vi "Take photo.vi"() -> ()   [LabVIEW 2020]
uses:
  <vilib>/userDefined/High Color/IMAQdx.ctl
  <vilib>/vision/driver/NI_Vision_Acquisition_Software.lvlib
  <vilib>/vision/NI_Vision_Development_Module.lvlib
panel:
  out "Number of Matches":i32
  out "error out":errorcluster
  out "Image 2":T1(plugin-control)
  in  "Parameters":T2={"Number of Matches Requested"=1, "Minimum Match Score"=800.0, "Angle Ranges"=[]}
  in  "File Path":path
  out "Image":T1(plugin-control)
  in  "stop":bool
  in  "Session In":T3
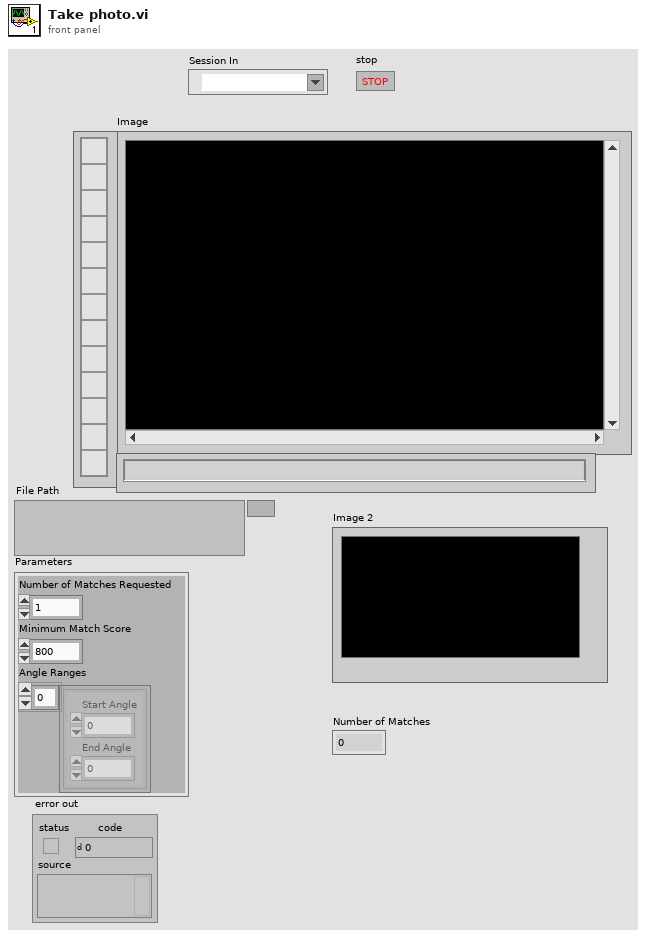
[diagram p1: front panel]
types:
  T1 = typedef "IMAQ Image.ctl" = refnum<image>
  T2 = cluster{"Number of Matches Requested":i32, "Minimum Match Score":sgl, "Angle Ranges":cluster{"Start Angle":sgl, "End Angle":sgl}[]}
  T3 = typedef "IMAQdx.ctl" = refnum<k21>
  T4 = cluster{"Position":cluster{"x":sgl, "y":sgl}, "Angle":sgl, "Scale":sgl, "Score":sgl, "Bounding Box":cluster{"x":sgl, "y":sgl}[]}[]
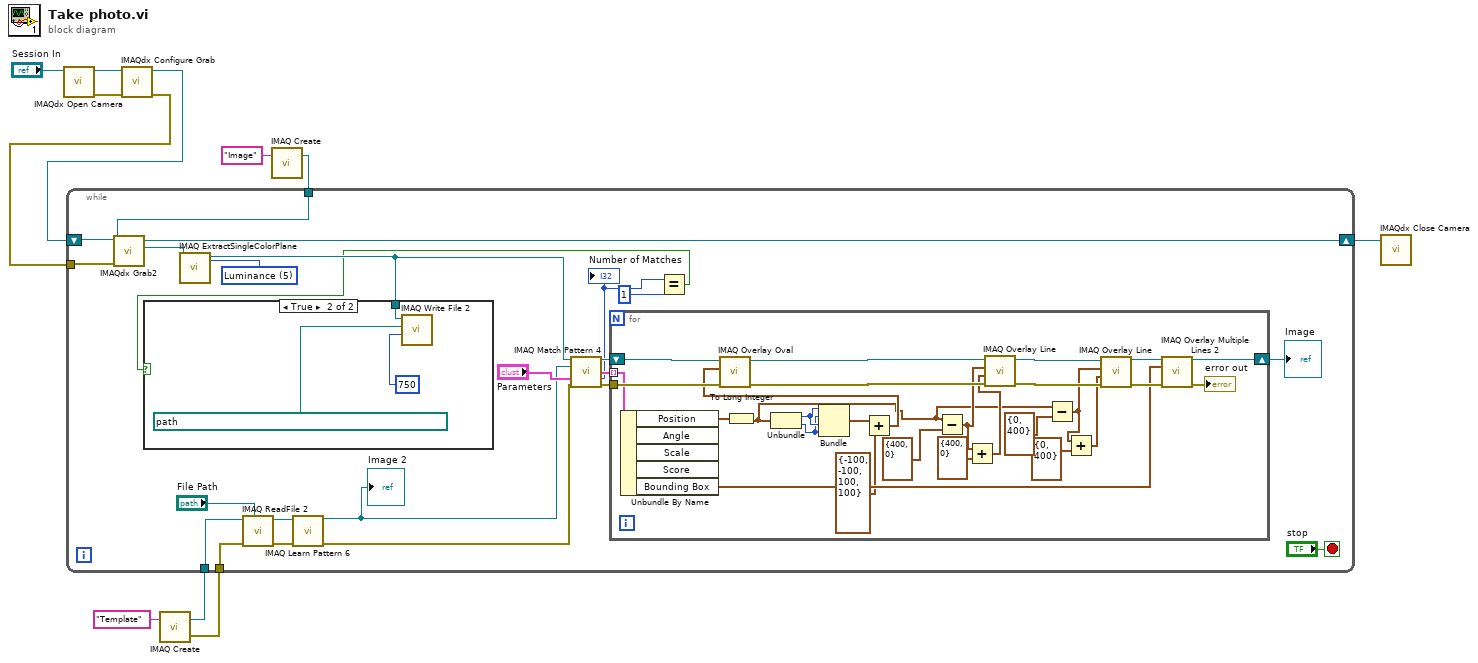
[diagram p0: block diagram]
diagram:
  n1 = call <vilib>:"IMAQdx Open Camera.vi"("Session In"="Session In") -> ("error out"=w10:errorcluster, "Session Out"=w9:T3)  [unwired: 9 in]
  n2 = call <vilib>:"IMAQdx Configure Grab.vi"("error in"=w10, "Session In"=w9) -> ("error out"=w6:errorcluster, "Session Out"=w7:T3)  [unwired: 8 in]
  n3 = call "IMAQ Create"("Image Name"="Template") -> ("New Image"=w2:T1, "error out"=w1:errorcluster)  [unwired: 4 in]
  n4 = call "IMAQ Create"("Image Name"="Image") -> ("New Image"=w4:T1)  [unwired: 4 in, 1 out]
  n5 = while {
    tunnel: w6 -> [w34]
    shift-right: [w33] -> w5
    shift-left: w7 -> [w30]
    tunnel: w4 -> [w31]
    tunnel: w2 -> [w27]
    tunnel: w1 -> [w26]
    stop <- "stop" stop-if-true
    w29 = 5 items=["Red", "Green", "Blue", "Hue", "Saturation", "Luminance", "Value", "Intensity"] ("Color Plane")
    n6 = call <vilib>:"IMAQdx Grab2.vi"("error in"=w34, "Image In"=w31, "Session In"=w30) -> ("Image Out"=w28:T1, "Session Out"=w33:T3)  [unwired: 5 in, 2 out]
    n7 = call "IMAQ ExtractSingleColorPlane"("Color Plane"=w29, "Image Src"=w28) -> ("Image Dst Out"=w22:T1)  [unwired: 2 in, 7 out]
    n8 = call "IMAQ ReadFile 2"("File Path"="File Path", "error in (no error)"=w26, "Image"=w27) -> ("error out"=w24:errorcluster, "Image Out"=w25:T1)  [unwired: 4 in, 3 out]
    n9 = call "IMAQ Learn Pattern 6"("Image"=w25, "error in (no error)"=w24) -> ("Template Image Out"=w20:T1, "error out"=w16:errorcluster)  [unwired: 11 in, 1 out]
    "Image 2" <- w20
    n10 = call "IMAQ Match Pattern 4"("Image"=w22, "Template Image"=w20, "Parameters"="Parameters", "error in (no error)"=w16) -> ("Image (duplicate)"=w19:T1, "Matches (real-world)"=w15:T4, "Number of Matches"=w14:i32, "error out"=w17:errorcluster)  [unwired: 7 in, 1 out]
    "Number of Matches" <- w14
    n11 = for {
      tunnel: w17 -> [w56]
      tunnel: w15 -> [w52] mode=indexing
      shift-right: [w57] -> w18
      shift-left: w19 -> [w61]
      n12 = Unbundle By Name(w52) -> ("Position"=w42:cluster{"x":sgl, "y":sgl}, "Bounding Box"=w49:cluster{"x":sgl, "y":sgl}[])  [unwired: 3 out]
      n13 = To Long Integer(number=w42) -> (32bit integer=w41:cluster{"x":i32, "y":i32})
      n14 = Unbundle(w41) -> ("x"=w51:i32, "y"=w50:i32)
      n15 = Bundle("x"=w51, "y"=w50, "x"=w51, "y"=w50) -> (w47:cluster{"x":i32, "y":i32, "x":i32, "y":i32})  [unwired: 1 in]
      n16 = Add(x=w47, y=cluster{"x":i32, "y":i32, "x":i32, "y":i32} {"x"=-100, "y"=-100, "x"=100, "y"=100}) -> (x+y=w46:cluster{"x":i32, "y":i32, "x":i32, "y":i32})
      n17 = call "IMAQ Overlay Oval"("error in (no error)"=w56, "Bounding Rectangle"=w46, "Image"=w61) -> ("error out"=w55:errorcluster, "Image Out"=w60:T1)  [unwired: 7 in]
      n18 = Subtract(x=w41, y=cluster{"x":i32, "y":i32} {"x"=400, "y"=0}) -> (x-y=w44:cluster{"x":i32, "y":i32})
      n19 = Add(x=w44, y=cluster{"x":i32, "y":i32} {"x"=400, "y"=0}) -> (x+y=w43:cluster{"x":i32, "y":i32})
      n20 = call "IMAQ Overlay Line"("error in (no error)"=w55, "End Point"=w43, "Start Point"=w44, "Image"=w60) -> ("error out"=w54:errorcluster, "Image Out"=w59:T1)  [unwired: 6 in]
      n21 = Subtract(x=w41, y=cluster{"x":i32, "y":i32} {"x"=0, "y"=400}) -> (x-y=w37:cluster{"x":i32, "y":i32})
      n22 = Add(x=w37, y=cluster{"x":i32, "y":i32} {"x"=0, "y"=400}) -> (x+y=w35:cluster{"x":i32, "y":i32})
      n23 = call "IMAQ Overlay Line"("error in (no error)"=w54, "End Point"=w35, "Start Point"=w37, "Image"=w59) -> ("error out"=w53:errorcluster, "Image Out"=w58:T1)  [unwired: 6 in]
      n24 = call "IMAQ Overlay Multiple Lines 2"("Image"=w58, "Line End Points"=w49, "error in (no error)"=w53) -> ("Image Out"=w57:T1, "error out"=→"error out":errorcluster)  [unwired: 11 in]
    }
    "Image" <- w18
    n25 = Equal?(x=w14, y=1) -> (x = y?=w12:bool)
    n26 = case shown="True" w12 {
      tunnel: w22 -> [_ w62]
      frame False {
      }
      frame True {
        n27 = call-poly "IMAQ Write File 2"("Image Quality"=u32 750, "File Path"=path "C:/Dane/Studia/SEM_6/OSP/Robienie zdjęcia/cos.jpg", "Image"=w62) -> ()  [unwired: 7 in, 2 out]
      }
    }
  }
  n28 = call <vilib>:"IMAQdx Close Camera.vi"("Session In"=w5) -> ()  [unwired: 10 in, 1 out]
